vi "test_InvalidEnumInConfig_ValidateMetadata_Error.vi"(8 "error in":errorcluster) -> (0 "error out":errorcluster, 2 "result":string, 3 "pass":bool)   [LabVIEW 2020, in "MeasurementServerTests.lvlib" / "Measurement Plugin Service Tests.lvlib"]
uses:
  Measurement Plugin Service Tests.lvlib
  Fake Measurement Plugin/Plugin VI and Control References.ctl
  Fake Measurement Plugin/Fake Measurement Plugin.lvclass
  C:/Dev/github/ni/measurementlink-labview/Source/Runtime/MeasurementLink Measurement Server/Measurement Plugin Service/Measurement Plugin Service.lvclass
  Measurement IO Enum Legal Characters.ctl
  Get Type Specializations Default.vi
  Measurement IO Enum Illegal Character Equal.ctl
  Runtime/MeasurementLink Measurement Server/Helpers/Error Strings Global Internal.vi
  Runtime/MeasurementLink Measurement Server/MeasurementLink Measurement Server.lvlib
  MeasurementServerTests.lvlib
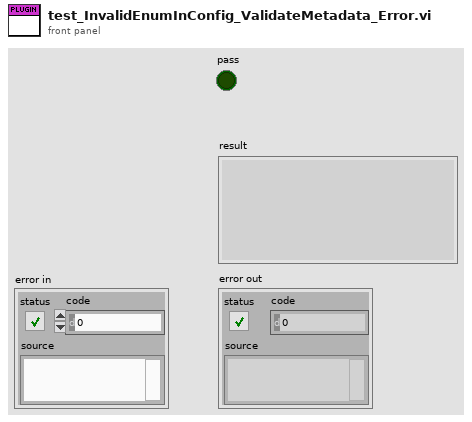
[diagram p1: front panel]
types:
  T1 = typedef "MeasurementServerTests.lvlib/Measurement Plugin Service Tests.lvlib/Fake Measurement Plugin.lvclass/Plugin VI and Control References.ctl" = cluster{"get measurement details VI ref":refnum<vi>, "get type specializations VI ref":refnum<vi>, "get UI details VI ref":refnum<vi>, "measurement logic VI ref":refnum<vi>, "measurement configuration ctl ref":refnum<vi>, "measurement results ctl path":refnum<vi>}
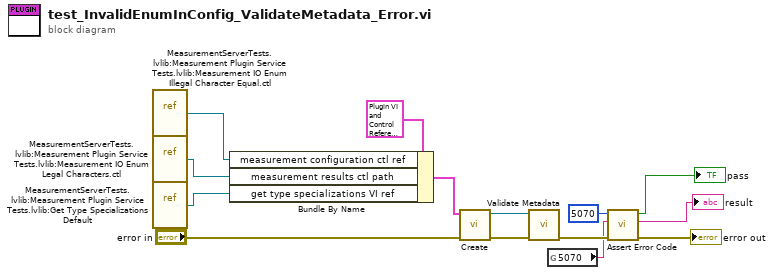
[diagram p0: block diagram]
diagram:
  n1 = vi-ref "MeasurementServerTests.lvlib:Measurement Plugin Service Tests.lvlib:Measurement IO Enum Illegal Character Equal.ctl"() -> (w7:refnum<vi>)
  n2 = vi-ref "MeasurementServerTests.lvlib:Measurement Plugin Service Tests.lvlib:Measurement IO Enum Legal Characters.ctl"() -> (w8:refnum<vi>)
  n3 = vi-ref "MeasurementServerTests.lvlib:Measurement Plugin Service Tests.lvlib:Get Type Specializations Default.vi"() -> (w12:refnum<vi>)
  n4 = Bundle By Name(cluster=T1 {"get measurement details VI ref"=refnum, "get type specializations VI ref"=refnum, "get UI details VI ref"=refnum, "measurement logic VI ref"=refnum, "measurement configuration ctl ref"=refnum, "measurement results ctl path"=refnum} ("plugin references"), "measurement configuration ctl ref"=w7, "measurement results ctl path"=w8, "get type specializations VI ref"=w12) -> (w9:T1)
  n5 = call "Create.vi"("error in"="error in", "plugin references"=w9) -> ("error out"=w11:errorcluster, "fake measurement plugin"=w14:refnum<class "Fake Measurement Plugin.lvclass">)  [unwired: 8 in]
  n6 = call "Validate Metadata.vi"("error in (no error)"=w11, "measurement plugin service in"=w14) -> ("error out"=w6:errorcluster)  [unwired: 8 in, 1 out]
  n7 = global read "Error Strings Global Internal.vi" "5070"() -> (w1:string)
  n8 = call "Assert Error Code.vi"("error in"=w6, "expected error description"=w1, "expected error code"=5070) -> ("error out"=→"error out":errorcluster, "details"=→"result":string, "error code match?"=→"pass":bool)  [unwired: 6 in]
